vi "Create GPIO Routes Array.vi"(11 "gpio route configurations":T1[](array[typedef]) {"Serial Channel" max=3 step=1}) -> (3 "gpio routes":i8[](array[numeric]))   [LabVIEW 2023, in "GettingStarted_Common_148X_Host.lvlib"]
uses:
  GettingStarted_Common_148X_Host.lvlib
  Types/GPIO Route Configuration.ctl
  Types/GPIO Route Direction.ctl
  Types/GPIO Route Line.ctl
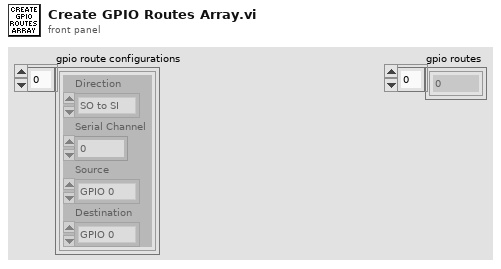
[diagram p1: front panel]
types:
  T1 = typedef "GettingStarted_Common_148X_Host.lvlib/GPIO Route Configuration.ctl" = cluster{"Direction":T2, "Serial Channel":u8, "Source":T3, "Destination":T3}
  T2 = typedef "GettingStarted_Common_148X_Host.lvlib/GPIO Route Direction.ctl" = enum8{"SO to SI", "SI to SO"}
  T3 = typedef "GettingStarted_Common_148X_Host.lvlib/GPIO Route Line.ctl" = enum16{"GPIO 0", "GPIO 1", "GPIO 2", "GPIO 3", "GPIO 4", "GPIO 5", "GPIO 6", "GPIO 7", "GPIO 8", "GPIO 9", "GPIO 10", "User"}
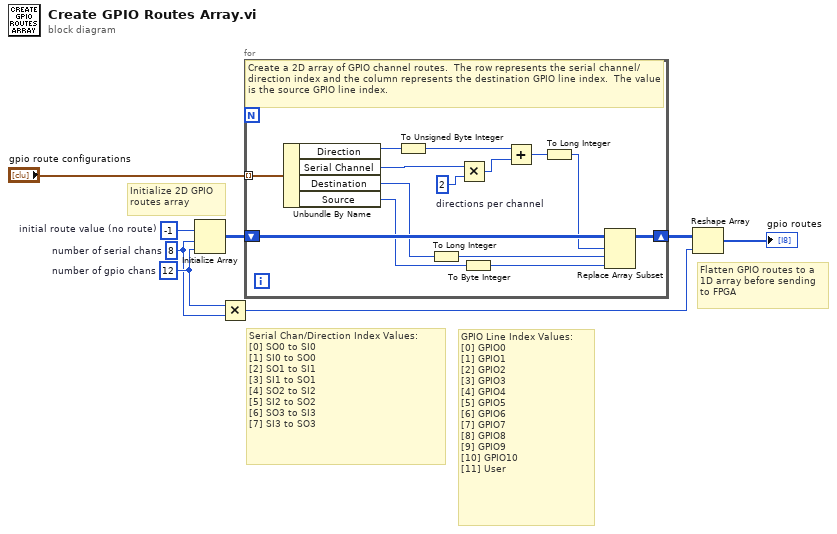
[diagram p0: block diagram]
diagram:
  w6 = 12  # number of gpio chans
  w5 = 8  # number of serial chans
  w1 = i8 -1  # initial route value (no route)
  # "GPIO Line Index Values:\n[0] GPIO0\n[1] GPIO1\n[2] GPIO2\n[3] GPIO3\n[4] GPIO4\n[5] GPIO5\n[6] GPIO6\n[7] GPIO7\n[8] GPIO8\n[9] GPIO9\n[10] GPIO10\n[11] User"
  # "Serial Chan/Direction Index Values:\n[0] SO0 to SI0\n[1] SI0 to SO0\n[2] SO1 to SI1\n[3] SI1 to SO1\n[4] SO2 to SI2\n[5] SI2 to SO2\n[6] SO3 to SI3\n[7] SI3 to SO3"
  # "Initialize 2D GPIO routes array"
  # "Flatten GPIO routes to a 1D array before sending to FPGA"
  n1 = Initialize Array(w1, w5, w6) -> (w3:i8[][])
  n2 = Multiply(x=w6, y=w5) -> (x*y=w7:i32)
  n3 = for {
    tunnel: "gpio route configurations" -> [w22] mode=indexing
    shift-right: [w10] -> w4
    shift-left: w3 -> [w14]
    w20 = u8 2  # directions per channel
    # "Create a 2D array of GPIO channel routes.  The row represents the serial channel/direction index and the column represents the destination GPIO line index.  The value is the source GPIO line index."
    n4 = Unbundle By Name(w22) -> ("Direction"=w19:T2, "Serial Channel"=w21:u8, "Destination"=w13:T3, "Source"=w9:T3)
    n5 = To Unsigned Byte Integer(number=w19) -> (unsigned 8bit integer=w18:u8)
    n6 = To Long Integer(number=w13) -> (32bit integer=w12:i32)
    n7 = Multiply(x=w21, y=w20) -> (x*y=w17:u8)
    n8 = To Byte Integer(number=w9) -> (8bit integer=w15:i8)
    n9 = Add(x=w18, y=w17) -> (x+y=w16:u8)
    n10 = To Long Integer(number=w16) -> (32bit integer=w11:i32)
    n11 = Replace Array Subset(array=w14, new element=w15, index (row)=w11, index (col)=w12) -> (w10:i8[][])
  }
  n12 = Reshape Array(w4, w7) -> (→"gpio routes":i8[])
